vi "FFID Setup.vi"(8 "Analysis Info cluster In":T1[](array[typedef]) {"Sync Delay Time (s)" format="%.4f"; "Total Meas Time (s)" format="%_5g"; "Sd Error in Variance" format="%_3g"; "Skew_u" format="%_3g"; "% u'/U" format="%_3g"; "Sd Error in Mean" format="%_3g"; "Kurt_u" format="%_3g"; "u^4" format="%_3g"; "u^3" format="%_3g"; "U" format="%_3g"; "u^2" format="%_3g"}) -> (0 "Analysis Info cluster Out":T1[](array[typedef]) {"Sync Delay Time (s)" format="%.4f"; "Total Meas Time (s)" format="%_5g"; "Sd Error in Variance" format="%_3g"; "Skew_u" format="%_3g"; "% u'/U" format="%_3g"; "Sd Error in Mean" format="%_3g"; "Kurt_u" format="%_3g"; "u^4" format="%_3g"; "u^3" format="%_3g"; "U" format="%_3g"; "u^2" format="%_3g"}, 3 "FFID Channels":bool)   [LabVIEW 2022 SP3]
uses:
  Controls/ok_button.ctl
  Controls/Analysis_info_cluster.ctl
  Controls/Inst_type.ctl
  Controls/Instrument_Array.ctl
  <vilib>/Utility/config.llb/Read Key (String).vi
  Globals/Meas_global.vi
  <vilib>/Utility/config.llb/NI_LVConfig.lvlib
panel:
  out "Message":string
  out "Measurement Setup Filename":string
  out "Comms Channel Number":i32
  in  "OK":T4
  in  "Control Unit":u16(ring) items=["129_Ch1", "129_Ch2", "163_Ch1", "163_Ch2"]
  in  "Sample Tube Size":u16(ring) items=["OD 0.51mm  ID 0.254mm", "OD 0.56mm  ID 0.305mm", "OD 0.81mm  ID 0.51mm", "OD 0.89mm  ID 0.584mm"]
  in  "Sample Tube Length (mm)":i32
  in  "Head Serial Number":u16(ring) items=["27", "05", "22", "13"]
  in  "FFID Type":u16(ring) items=["HFR400", "HFR500"]
  out "Channel Name":string
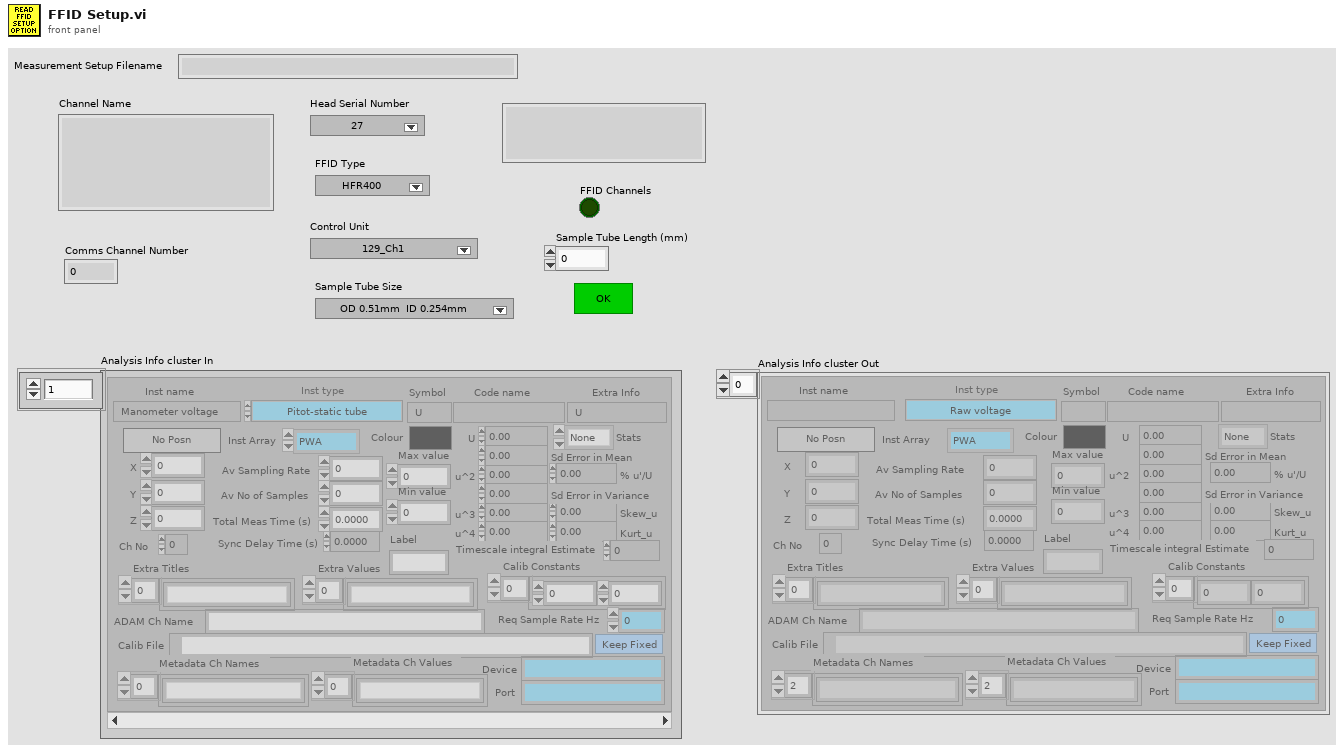
[diagram p1: front panel]
types:
  T1 = typedef "Analysis_info_cluster.ctl" = cluster{"Colour":u32, "Inst type":T2, "Inst name":string, "Symbol":string, "Code name":string, "Extra Info":string, "Inst Array":T3, "Extra Titles":string[], "Extra Values":string[], "U":dbl, "u^2":dbl, "u^3":dbl, "u^4":dbl, "Skew_u":dbl, "Kurt_u":dbl, "Sd Error in Mean":dbl, "% u'/U":dbl, "X":dbl, "Y":dbl, "Z":dbl, "Timescale integral Estimate":dbl, "Sd Error in Variance":dbl, "Calib File":path, "Calib Constants":dbl[], "Output Position":bool, "Stats":enum16{"None", "Basic", "Full"}, "Av Sampling Rate":dbl, "Av No of Samples":dbl, "Total Meas Time (s)":dbl, "ADAM Ch Name":string, "Max value":dbl, "Min value":dbl, "Req Sample Rate Hz":dbl, "Sync Delay Time (s)":dbl, "Ch No":i16, "Device":string, "Use Latest Calib":bool, "Port":string, "Metadata Ch Names":string[], "Metadata Ch Values":string[], "Label":string}
  T2 = typedef "Inst_type.ctl" = enum16{"Raw voltage", "Raw with zero offsetting", "Propeller anemometer", "Pressure Transducer", "Pitot-static tube", "Hot wire", "Cross wire 1", "Cross wire 2", "Generic Linear", "Generic Polynomial", "Generic BackPoly", "Fast FID", "Thermocouple", "Cold wire", "Pulsed Wire", "LDA Vel", "LDA Tran time", "LDA Arr time", "Microphone"}
  T3 = typedef "Instrument_Array.ctl" = enum16{"PWA", "LDA", "Analogue"}
  T4 = typedef "ok_button.ctl" = bool
  T5 = typedef "NI_LVConfig.lvlib/Config Data RefNum.ctl" = refnum<k1>
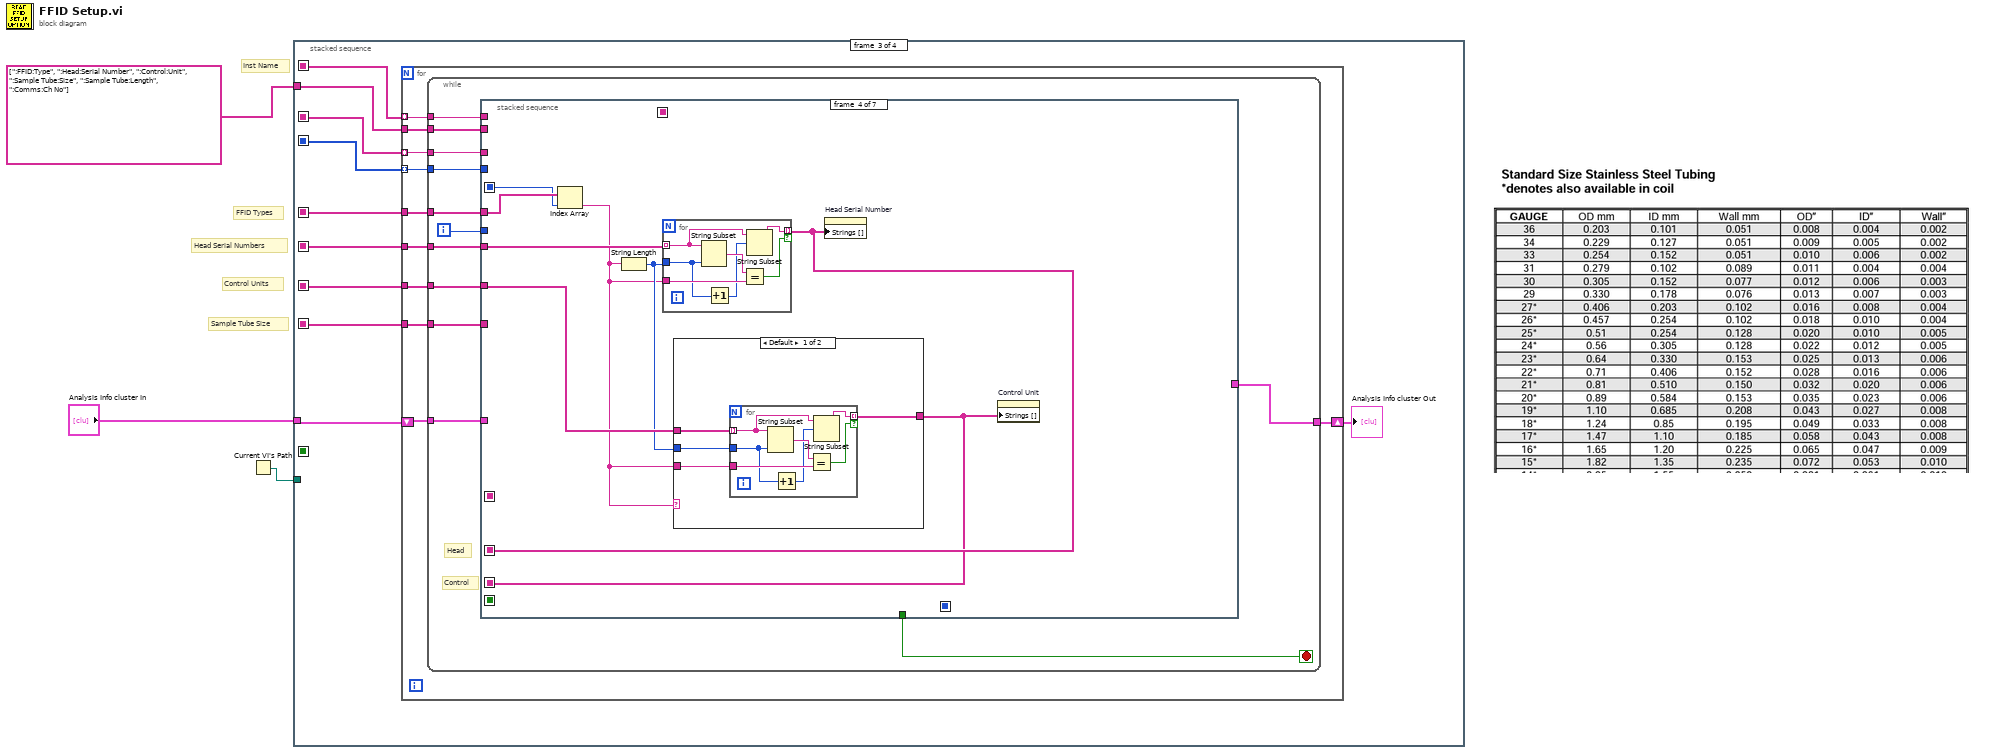
[diagram p0: block diagram]
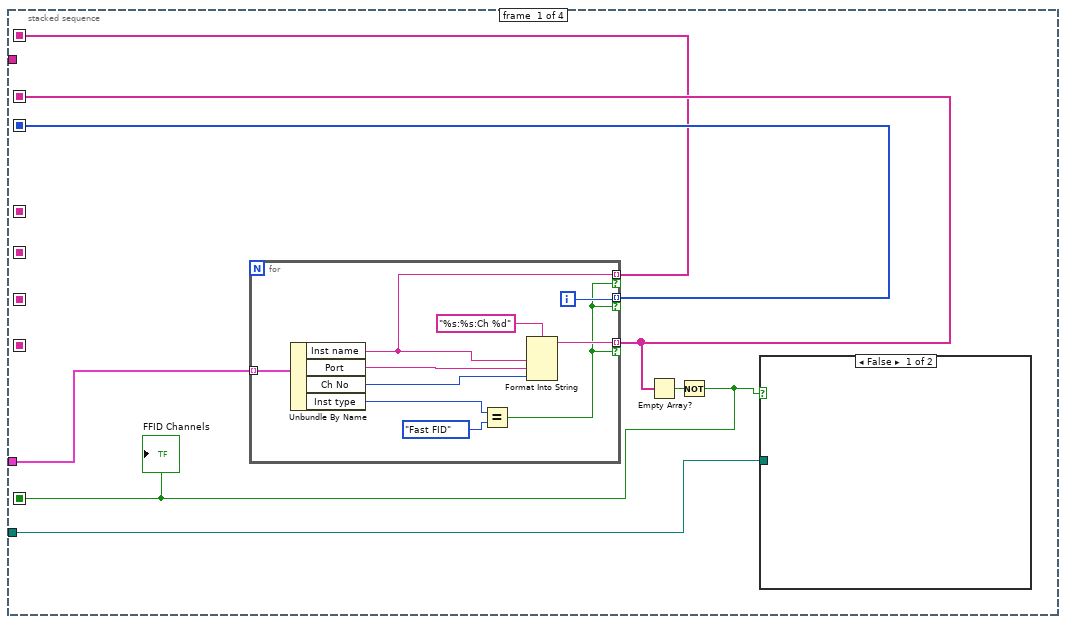
[diagram p2: hidden frame]
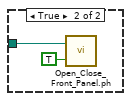
[diagram p3: hidden frame]
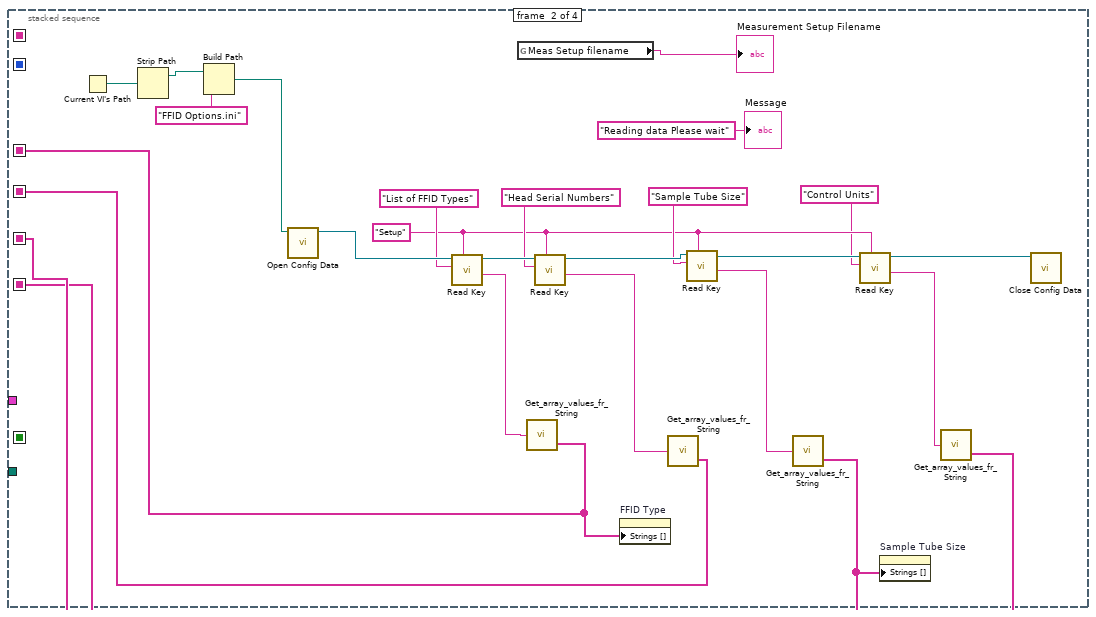
[diagram p4: hidden frame]
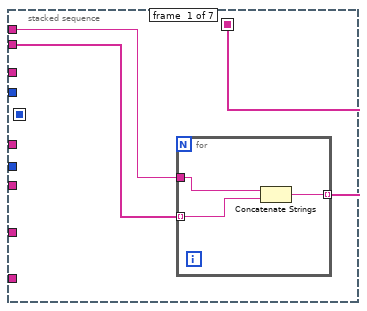
[diagram p5: hidden frame]
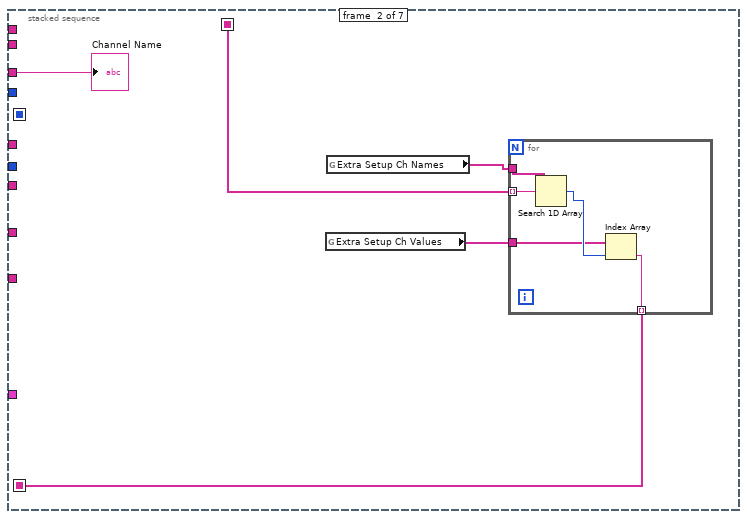
[diagram p6: hidden frame]
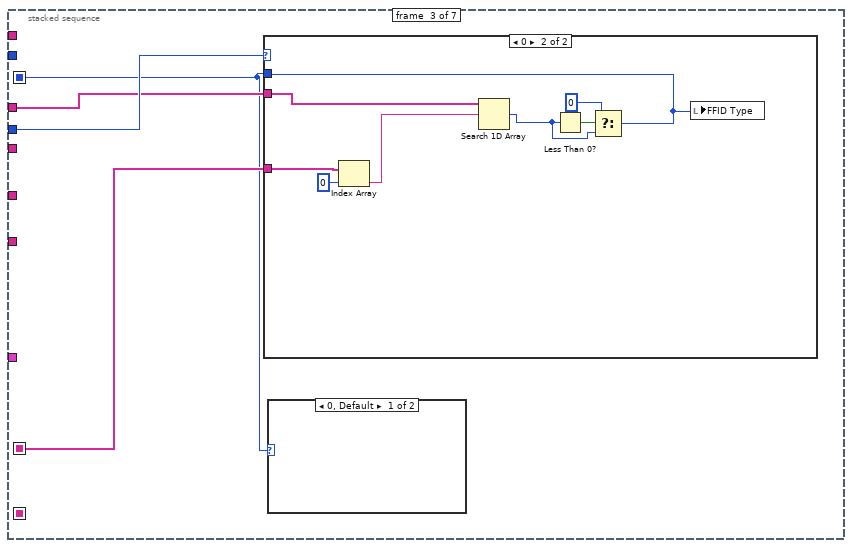
[diagram p7: hidden frame]
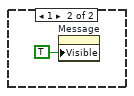
[diagram p8: hidden frame]
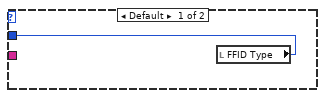
[diagram p9: hidden frame]
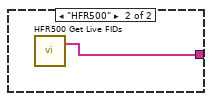
[diagram p10: hidden frame]
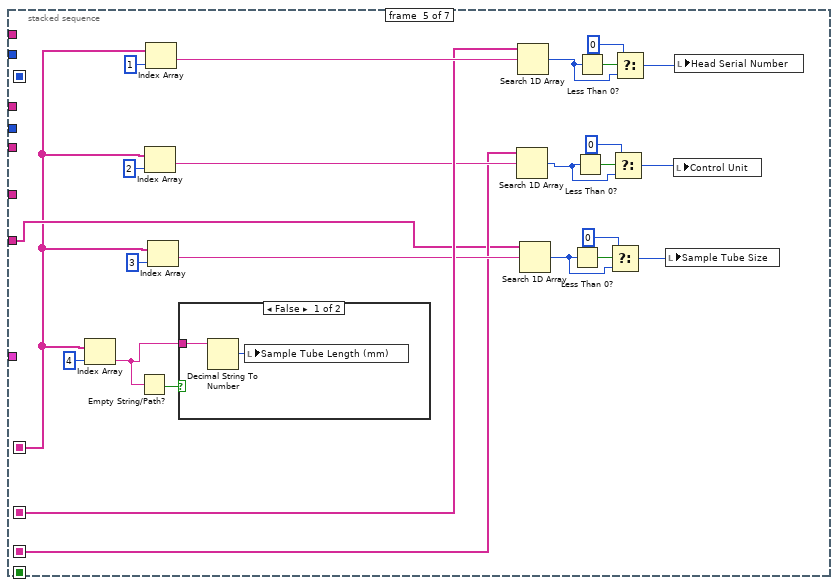
[diagram p11: hidden frame]
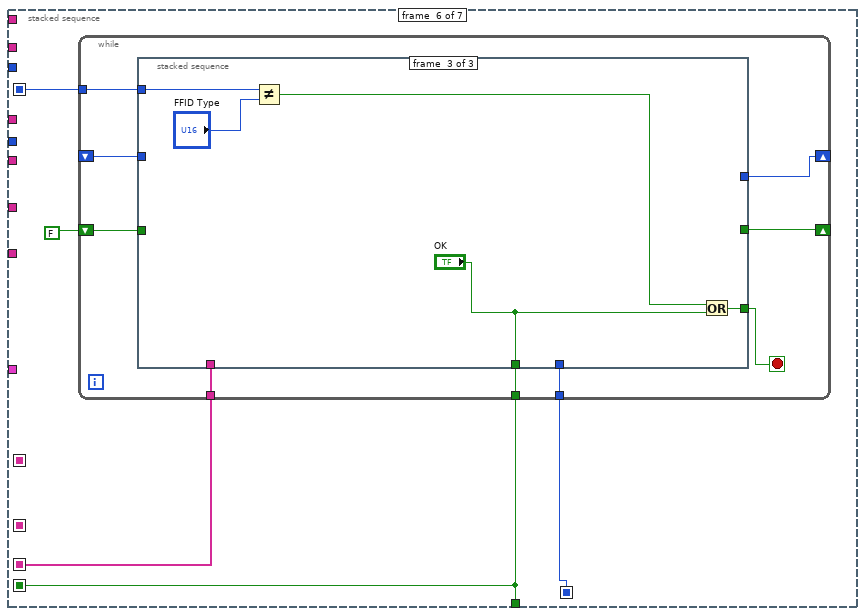
[diagram p13: hidden frame]
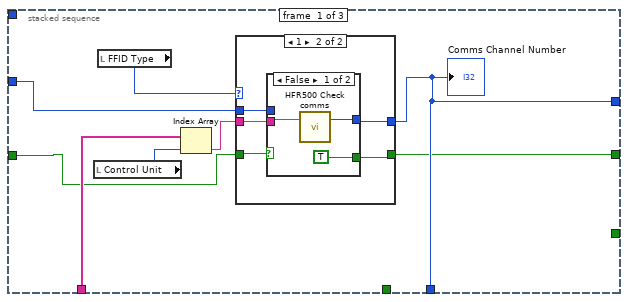
[diagram p14: hidden frame]
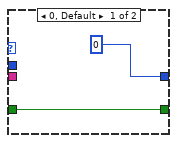
[diagram p15: hidden frame]
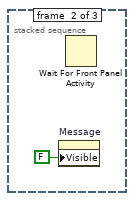
[diagram p17: hidden frame]
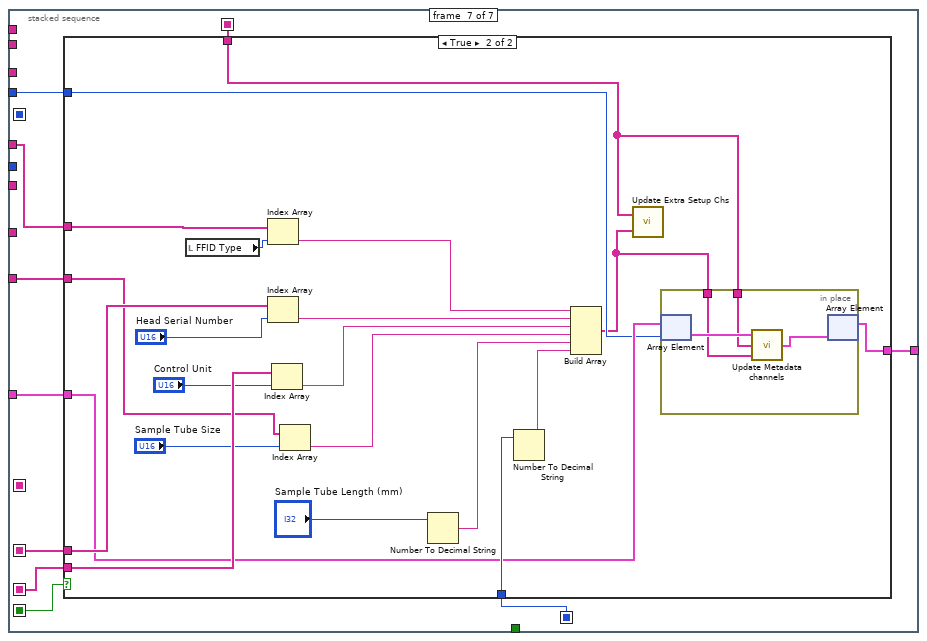
[diagram p18: hidden frame]
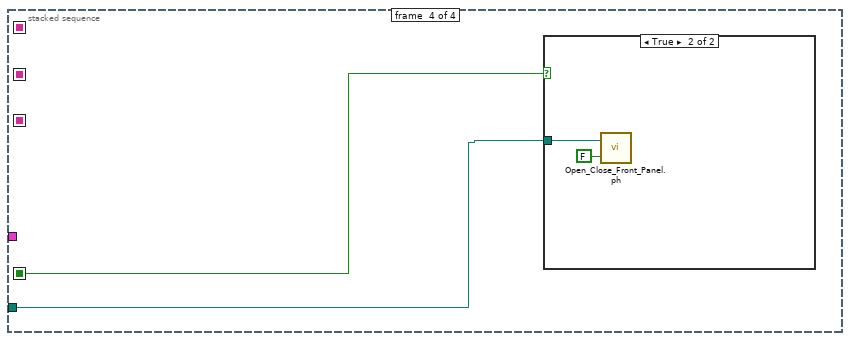
[diagram p20: hidden frame]
diagram:
  # "Inst Name"
  # "Control Units"
  # "Sample Tube Size"
  # "Head Serial Numbers"
  # "FFID Types"
  n1 = Current VI's Path() -> (path=w1:path)
  n2 = stacked-sequence {
    seq-local: [w8 _ _ _] -> [_ _ w56 _]
    seq-local: [_ w30 _ _] -> [_ _ w53 _]
    seq-local: [_ w32 _ _] -> [_ _ w52 _]
    seq-local: [_ w29 _ _] -> [_ _ w50 _]
    seq-local: [_ w31 _ _] -> [_ _ w51 _]
    seq-local: [w9 _ _ _] -> [_ _ w55 _]
    seq-local: [w5 _ _ _] -> [_ _ _ w239]
    seq-local: [w4 _ _ _] -> [_ _ w47 _]
    tunnel: "Analysis Info cluster In" -> [w10 _ w49 _]
    tunnel: string[] [":FFID:Type", ":Head:Serial Number", ":Control:Unit", ":Sample Tube:Size", ":Sample Tube:Length", ":Comms:Ch No"] -> [_ _ w54 _]
    tunnel: w1 -> [w7 _ _ w240]
    frame #0 {
      n3 = for {
        tunnel: w10 -> [w19] mode=indexing
        tunnel: [w16] -> w8 mode=indexing if=w13
        tunnel: [w15] -> w9 mode=indexing if=w13
        tunnel: [w14] -> w4 mode=indexing if=w13
        i -> [w15]
        n4 = Unbundle By Name(w19) -> ("Inst name"=w14:string, "Port"=w21:string, "Ch No"=w20:i16, "Inst type"=w17:T2)
        n5 = Equal?(x=w17, y=Inst_type."Fast FID" ("Inst type")) -> (x = y?=w13:bool)
        n6 = Format Into String(format string="%s:%s:Ch %d", w14, w21, w20) -> (resulting string=w16:string)  [unwired: 2 in, 1 out]
      }
      n7 = Empty Array?(array=w8) -> (empty?=w6:bool)
      n8 = Not(x=w6) -> (.not. x?=w5:bool)
      "FFID Channels" <- w5
      n9 = case shown="False" w5 {
        tunnel: w7 -> [_ w12]
        frame False {
        }
        frame True {
          n10 = call "Open_Close_Front_Panel.ph.vi"("openWindow (T)"=TRUE, "VI path"=w12) -> ()  [unwired: 1 in, 1 out]
        }
      }
    }
    frame #1 {
      w38 = "Setup" ("section")
      n11 = Current VI's Path() -> (path=w28:path)
      n12 = Strip Path(path=w28) -> (stripped path=w27:path)  [unwired: 1 out]
      n13 = Build Path(base path=w27, name or relative path="FFID Options.ini") -> (appended path=w25:path)
      n14 = call <vilib>:"Open Config Data.vi"("configuration file path"=w25) -> ("refnum"=w46:T5)  [unwired: 8 in, 2 out]
      n15 = call-poly <vilib>:"Read Key.vi"("section"=w38, "key"="List of FFID Types", "refnum"=w46) -> ("value"=w40:string, "refnum out"=w43:T5)  [unwired: 5 in, 2 out]
      n16 = global read "Meas_global.vi" "Meas Setup filename"() -> (→"Measurement Setup Filename":string)
      n17 = call "Get_array_values_fr_String.vi"("String Value"=w40) -> ("String array"=w30:string[])  [unwired: 1 out]
      n18 = call-poly <vilib>:"Read Key.vi"("section"=w38, "key"="Head Serial Numbers", "refnum"=w43) -> ("value"=w39:string, "refnum out"=w44:T5)  [unwired: 5 in, 2 out]
      n19 = property on="FFID Type" class="Ring (strict)"("Strings []"=w30) -> ()  [unwired: 2 in, 2 out]
      n20 = call "Get_array_values_fr_String.vi"("String Value"=w39) -> ("String array"=w32:string[])  [unwired: 1 out]
      n21 = call-poly <vilib>:"Read Key.vi"("section"=w38, "key"="Sample Tube Size", "refnum"=w44) -> ("value"=w33:string, "refnum out"=w37:T5)  [unwired: 5 in, 2 out]
      n22 = call "Get_array_values_fr_String.vi"("String Value"=w33) -> ("String array"=w29:string[])  [unwired: 1 out]
      n23 = call-poly <vilib>:"Read Key.vi"("section"=w38, "key"="Control Units", "refnum"=w37) -> ("value"=w34:string, "refnum out"=w36:T5)  [unwired: 5 in, 2 out]
      n24 = property on="Sample Tube Size" class="Ring (strict)"("Strings []"=w29) -> ()  [unwired: 2 in, 2 out]
      n25 = call "Get_array_values_fr_String.vi"("String Value"=w34) -> ("String array"=w31:string[])  [unwired: 1 out]
      n26 = call <vilib>:"Close Config Data.vi"("refnum"=w36) -> ()  [unwired: 9 in, 2 out]
      "Message" <- "Reading data Please wait" ("Reading data Please wait")
    }
    frame #2 {
      n27 = for {
        tunnel: w56 -> [w66] mode=indexing
        tunnel: w55 -> [w65] mode=indexing
        tunnel: w54 -> [w64]
        tunnel: w53 -> [w63]
        tunnel: w52 -> [w62]
        tunnel: w51 -> [w61]
        tunnel: w50 -> [w60]
        shift-right: [w58] -> w48
        shift-left: w49 -> [w59]
        tunnel: w47 -> [w57] mode=indexing
        n28 = while {
          tunnel: w66 -> [w78]
          tunnel: w59 -> [w77]
          tunnel: w65 -> [w76]
          tunnel: w64 -> [w75]
          tunnel: w63 -> [w74]
          tunnel: w62 -> [w73]
          tunnel: w61 -> [w72]
          tunnel: w60 -> [w71]
          tunnel: [w69] -> w58
          tunnel: w57 -> [w67]
          i -> [w68]
          stop <- w70 stop-if-true
          # "Control"
          # "Head"
          n29 = stacked-sequence {
            seq-local: [_ w88 _ _ _ _ _] -> [_ _ w97 _ w150 _ _]
            seq-local: [_ _ _ w112 _ _ _] -> [_ _ _ _ w158 _ w207]
            seq-local: [_ _ _ w110 _ _ _] -> [_ _ _ _ w153 w165 w206]
            seq-local: [_ _ w95 _ _ _ _] -> [_ _ _ w111 _ w167 _]
            seq-local: [_ _ _ _ _ w166 _] -> [_ _ _ _ _ _ w212]
            seq-local: [w79 _ _ _ _ _ _] -> [_ w87 _ _ _ _ w204]
            seq-local: [_ _ _ _ _ w164 _] -> [_ _ _ _ _ _ w203]
            tunnel: w78 -> [_ w89 _ _ _ _ _]
            tunnel: w77 -> [_ _ _ _ _ _ w210]
            tunnel: w76 -> [_ _ _ _ _ _ w211]
            tunnel: w75 -> [w80 _ _ _ _ _ _]
            tunnel: w74 -> [_ _ w96 w115 _ _ w208]
            tunnel: w73 -> [_ _ _ w113 _ _ _]
            tunnel: w72 -> [_ _ _ w116 _ _ _]
            tunnel: w71 -> [_ _ _ _ w152 _ w205]
            tunnel: [_ _ _ _ _ w166 _] -> w70
            tunnel: [_ _ _ _ _ _ w209] -> w69
            tunnel: w68 -> [_ _ w98 _ _ _ _]
            tunnel: w67 -> [w81 _ _ _ _ _ _]
            frame #0 {
              n30 = for {
                tunnel: w81 -> [w84]
                tunnel: w80 -> [w83] mode=indexing
                tunnel: [w82] -> w79 mode=indexing
                n31 = Concatenate Strings(w84, w83) -> (w82:string)
              }
            }
            frame #1 {
              n32 = global read "Meas_global.vi" "Extra Setup Ch Values"() -> (w85:string[])
              n33 = global read "Meas_global.vi" "Extra Setup Ch Names"() -> (w86:string[])
              n34 = for {
                tunnel: w87 -> [w94] mode=indexing
                tunnel: [w92] -> w88 mode=indexing
                tunnel: w86 -> [w91]
                tunnel: w85 -> [w90]
                n35 = Search 1D Array(1D array=w91, element=w94) -> (index of element=w93:i32)  [unwired: 1 out]
                n36 = Index Array(array=w90, index=w93) -> (element=w92:string)
              }
              "Channel Name" <- w89
            }
            frame #2 {
              n37 = case shown="0" w98 {
                tunnel: [w100 w101] -> w95
                tunnel: w97 -> [_ w104]
                tunnel: w96 -> [_ w102]
                frame Default {
                  n38 = local read "FFID Type"() -> (w100:u16)
                }
                frame 0 {
                  n39 = Index Array(array=w104, index=0) -> (element=w103:string)
                  n40 = Search 1D Array(1D array=w102, element=w103) -> (index of element=w106:i32)  [unwired: 1 out]
                  n41 = Less Than 0?(x=w106) -> (x < 0?=w108:bool)
                  n42 = Select(t=0, s=w108, f=w106) -> (s? t:f=w101:i32)
                  n43 = local write "FFID Type"(w101) -> ()
                }
              }
              n44 = case shown="0, Default" w95 {
                frame 0, Default {
                }
                frame 1 {
                  n45 = property on="Message" class="Str"("Visible"=TRUE) -> ()  [unwired: 2 in, 2 out]
                }
              }
            }
            frame #3 {
              n46 = Index Array(array=w115, index=w111) -> (element=w109:string)
              n47 = String Length(string=w109) -> (length=w114:i32)
              n48 = for {
                tunnel: w114 -> [w130]
                tunnel: w113 -> [w132] mode=indexing
                tunnel: w109 -> [w134]
                tunnel: [w131] -> w112 mode=indexing if=w133
                n49 = String Subset(string=w132, length (rest)=w130) -> (substring=w135:string)  [unwired: 1 in]
                n50 = Increment(x=w130) -> (x+1=w129:i32)
                n51 = Equal?(x=w135, y=w134) -> (x = y?=w133:bool)
                n52 = String Subset(string=w132, offset (0)=w129) -> (substring=w131:string)  [unwired: 1 in]
              }
              n53 = case shown="Default" w109 {
                tunnel: w116 -> [w120 _]
                tunnel: w114 -> [w119 _]
                tunnel: w109 -> [w118 _]
                tunnel: [w117 w128] -> w110
                frame Default {
                  n54 = for {
                    tunnel: w119 -> [w122]
                    tunnel: w120 -> [w124] mode=indexing
                    tunnel: w118 -> [w126]
                    tunnel: [w123] -> w117 mode=indexing if=w125
                    n55 = String Subset(string=w124, length (rest)=w122) -> (substring=w127:string)  [unwired: 1 in]
                    n56 = Increment(x=w122) -> (x+1=w121:i32)
                    n57 = Equal?(x=w127, y=w126) -> (x = y?=w125:bool)
                    n58 = String Subset(string=w124, offset (0)=w121) -> (substring=w123:string)  [unwired: 1 in]
                  }
                }
                frame "HFR500" {
                  n59 = call "HFR500 Get Live FIDs.vi"() -> ("Available Channels"=w128:string[])  [unwired: 3 in]
                }
              }
              n60 = property on="Head Serial Number" class="Ring (strict)"("Strings []"=w112) -> ()  [unwired: 2 in, 2 out]
              n61 = property on="Control Unit" class="Ring (strict)"("Strings []"=w110) -> ()  [unwired: 2 in, 2 out]
            }
            frame #4 {
              n62 = Index Array(array=w150, index=4) -> (element=w149:string)
              n63 = Empty String/Path?(string/path=w149) -> (empty?=w148:bool)
              n64 = Index Array(array=w150, index=2) -> (element=w157:string)
              n65 = Index Array(array=w150, index=1) -> (element=w159:string)
              n66 = Index Array(array=w150, index=3) -> (element=w154:string)
              n67 = case shown="False" w148 {
                tunnel: w149 -> [w161 _]
                frame False {
                  n68 = Decimal String To Number(string=w161) -> (number=w162:i32)  [unwired: 2 in, 1 out]
                  n69 = local write "Sample Tube Length (mm)"(w162) -> ()
                }
                frame True {
                }
              }
              n70 = Search 1D Array(1D array=w153, element=w157) -> (index of element=w139:i32)  [unwired: 1 out]
              n71 = Search 1D Array(1D array=w158, element=w159) -> (index of element=w138:i32)  [unwired: 1 out]
              n72 = Search 1D Array(1D array=w152, element=w154) -> (index of element=w146:i32)  [unwired: 1 out]
              n73 = Less Than 0?(x=w146) -> (x < 0?=w147:bool)
              n74 = Less Than 0?(x=w139) -> (x < 0?=w142:bool)
              n75 = Less Than 0?(x=w138) -> (x < 0?=w141:bool)
              n76 = Select(t=0, s=w147, f=w146) -> (s? t:f=w144:i32)
              n77 = Select(t=0, s=w142, f=w139) -> (s? t:f=w136:i32)
              n78 = Select(t=0, s=w141, f=w138) -> (s? t:f=w137:i32)
              n79 = local write "Sample Tube Size"(w144) -> ()
              n80 = local write "Control Unit"(w136) -> ()
              n81 = local write "Head Serial Number"(w137) -> ()
            }
            frame #5 {
              n82 = while {
                tunnel: w167 -> [w176]
                tunnel: [w174] -> w166
                shift-right: [w168] -> _
                shift-left: FALSE -> [w171]
                tunnel: w165 -> [w173]
                tunnel: [w172] -> w164
                shift-right: [w169] -> _
                shift-left: _ -> [w170]
                stop <- w175 stop-if-true
                n83 = stacked-sequence {
                  tunnel: w176 -> [_ _ w202]
                  tunnel: [_ _ w200] -> w175
                  tunnel: [_ _ "OK"] -> w174
                  tunnel: w173 -> [w184 _ _]
                  tunnel: [w182 _ _] -> w172
                  tunnel: w171 -> [w183 _ _]
                  tunnel: w170 -> [w177 _ _]
                  tunnel: [w182 _ _] -> w169
                  tunnel: [w181 _ _] -> w168
                  frame #0 {
                    n84 = local read "Control Unit"() -> (w178:u16)
                    n85 = local read "FFID Type"() -> (w180:u16)
                    n86 = Index Array(array=w184, index=w178) -> (element=w179:string)
                    n87 = case shown="1" w180 {
                      tunnel: w179 -> [_ w191]
                      tunnel: [0 ("Comms Channel Number") w190] -> w182
                      tunnel: [w185 w189] -> w181
                      tunnel: w183 -> [w185 w188]
                      tunnel: w177 -> [_ w187]
                      frame 0, Default {
                      }
                      frame 1 {
                        n88 = case shown="False" w188 {
                          selector: w188 -> [_ w196]
                          tunnel: w191 -> [w194 _]
                          tunnel: [w193 w195] -> w190
                          tunnel: [TRUE w196] -> w189
                          tunnel: w187 -> [_ w195]
                          frame False {
                            n89 = call "HFR500 Check comms.vi"("Channel Name String"=w194) -> ("Comms Channel Number"=w193:i32)  [unwired: 2 in]
                          }
                          frame True {
                          }
                        }
                      }
                    }
                    "Comms Channel Number" <- w182
                  }
                  frame #1 {
                    n90 = property on="Message" class="Str"("Visible"=FALSE) -> ()  [unwired: 2 in, 2 out]
                    n91 = Wait For Front Panel Activity() -> ()  [unwired: 3 in, 1 out]
                  }
                  frame #2 {
                    n92 = Not Equal?(x=w202, y="FFID Type") -> (x != y?=w201:bool)
                    n93 = Or(x=w201, y="OK") -> (x .or. y?=w200:T4)
                  }
                }
              }
            }
            frame #6 {
              n94 = case shown="True" w212 {
                tunnel: w211 -> [_ w217]
                tunnel: w210 -> [w213 w218]
                tunnel: [w213 w214] -> w209
                tunnel: w208 -> [_ w234]
                tunnel: w207 -> [_ w230]
                tunnel: w206 -> [_ w228]
                tunnel: w205 -> [_ w224]
                tunnel: w204 -> [_ w216]
                tunnel: w203 -> [_ w220]
                frame False {
                }
                frame True {
                  n95 = local read "FFID Type"() -> (w233:u16)
                  n96 = Index Array(array=w234, index=w233) -> (element=w232:string)
                  n97 = Index Array(array=w230, index="Head Serial Number") -> (element=w229:string)
                  n98 = Index Array(array=w228, index="Control Unit") -> (element=w226:string)
                  n99 = Index Array(array=w224, index="Sample Tube Size") -> (element=w223:string)
                  n100 = Number To Decimal String(number="Sample Tube Length (mm)") -> (decimal integer string=w221:string)  [unwired: 1 in]
                  n101 = Number To Decimal String(number=w220) -> (decimal integer string=w219:string)  [unwired: 1 in]
                  n102 = Build Array(w232, w229, w226, w223, w221, w219) -> (w215:string[])
                  n103 = call "Update Extra Setup Chs.vi"("Extra Ch Values"=w215, "Extra Ch Names"=w216) -> ()  [unwired: 2 in]
                  n104 = in-place {
                    in-place-border: w216 -> [w237]
                    in-place-border: w215 -> [w236]
                    n105 = in-place-array #1(w218, w217) -> (w238:T1)
                    n106 = call "Update Metadata channels.vi"("Metadata Values"=w236, "Metadata Names"=w237, "Analysis info Cluster in"=w238) -> ("Analysis info Cluster out"=w235:T1)
                    n107 = in-place-array #1(w235) -> (w214:T1[])  [unwired: 1 out]
                  }
                }
              }
            }
          }
        }
      }
      "Analysis Info cluster Out" <- w48
    }
    frame #3 {
      n108 = case shown="True" w239 {
        tunnel: w240 -> [_ w242]
        frame False {
        }
        frame True {
          n109 = call "Open_Close_Front_Panel.ph.vi"("openWindow (T)"=FALSE, "VI path"=w242) -> ()  [unwired: 1 in, 1 out]
        }
      }
    }
  }
